vi "get values from a control in a cluster using reference.vi"(9 "names":string[](array[string]), 11 "Clust Refnum":refnum<vi>) -> (2 "Values":variant)   [LabVIEW 2015]
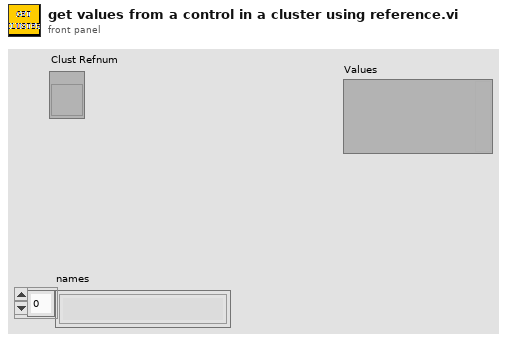
[diagram p1: front panel]
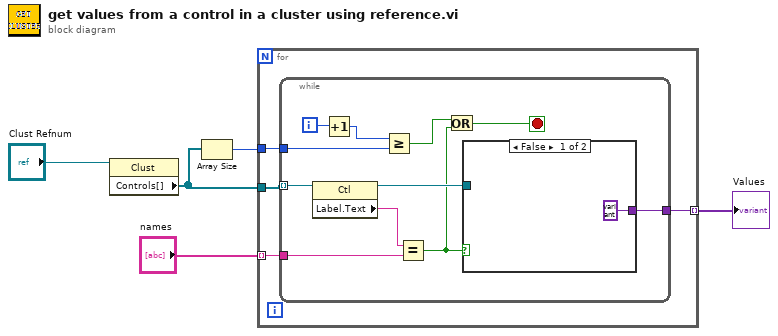
[diagram p0: block diagram]
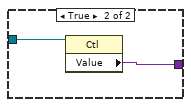
[diagram p2: hidden frame]
diagram:
  n1 = property class="Clust"(reference="Clust Refnum") -> ("Controls[]"=w3:refnum<vi>[])  [unwired: 1 in, 2 out]
  n2 = Array Size(array=w3) -> (size(s)=w1:i32)
  n3 = for {
    tunnel: "names" -> [w8] mode=indexing
    tunnel: w3 -> [w9]
    tunnel: [w7] -> w2 mode=indexing
    tunnel: w1 -> [w6]
    n4 = while {
      tunnel: w9 -> [w20] mode=indexing
      tunnel: w8 -> [w19]
      tunnel: w6 -> [w12]
      tunnel: [w15] -> w7
      i -> [w11]
      stop <- w18 stop-if-true
      n5 = property class="Ctl"(reference=w20) -> (reference out=w16:refnum<vi>, "Label.Text"=w17:string)  [unwired: 1 in, 1 out]
      n6 = Increment(x=w11) -> (x+1=w10:i32)
      n7 = Greater Or Equal?(x=w10, y=w12) -> (x >= y?=w14:bool)
      n8 = Equal?(x=w17, y=w19) -> (x = y?=w13:bool)
      n9 = Or(x=w14, y=w13) -> (x .or. y?=w18:bool)
      n10 = case shown="False" w13 {
        tunnel: w16 -> [_ w23]
        tunnel: [variant ("Value") w22] -> w15
        frame False {
        }
        frame True {
          n11 = property class="Ctl"(reference=w23) -> ("Value"=w22:variant)  [unwired: 1 in, 2 out]
        }
      }
    }
  }
  "Values" <- w2
